vi "test variant to json uint.vi"(8 "error in (no error)":errorcluster) -> (0 "error out":errorcluster)   [LabVIEW 2019, in "labview_json_tests.lvlib"]
uses:
  labview_json_tests.lvlib
  lib/labview_json.lvlib
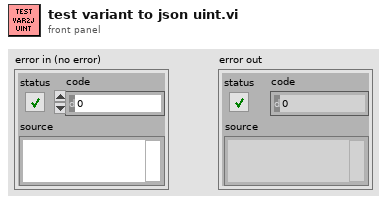
[diagram p1: front panel]
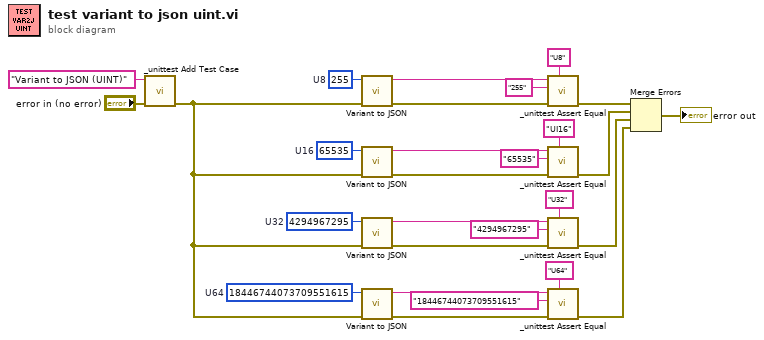
[diagram p0: block diagram]
diagram:
  w13 = u64 18446744073709551615  # U64
  w12 = u32 4294967295  # U32
  w14 = u16 65535  # U16
  w15 = u8 255  # U8
  n1 = call "_unittest Add Test Case.vi"("error in (no error)"="error in (no error)", "Test Case"="Variant to JSON (UINT)") -> ("error out"=w3:errorcluster)  [unwired: 9 in]
  n2 = call "Variant to JSON.vi"("error in (no error)"=w3, "Variant in"=w15) -> ("error out"=w21:errorcluster, "JSON"=w20:string)  [unwired: 8 in]
  n3 = call "Variant to JSON.vi"("error in (no error)"=w3, "Variant in"=w14) -> ("error out"=w19:errorcluster, "JSON"=w18:string)  [unwired: 8 in]
  n4 = call "Variant to JSON.vi"("error in (no error)"=w3, "Variant in"=w12) -> ("error out"=w6:errorcluster, "JSON"=w7:string)  [unwired: 8 in]
  n5 = call "Variant to JSON.vi"("error in (no error)"=w3, "Variant in"=w13) -> ("error out"=w8:errorcluster, "JSON"=w9:string)  [unwired: 8 in]
  n6 = call "_unittest Assert Equal.vi"("Message"="U8", "error in (no error)"=w21, "Expected Value"="255", "Actual Value"=w20) -> ("error out"=w26:errorcluster)  [unwired: 7 in]
  n7 = call "_unittest Assert Equal.vi"("Message"="UI16", "error in (no error)"=w19, "Expected Value"="65535", "Actual Value"=w18) -> ("error out"=w22:errorcluster)  [unwired: 7 in]
  n8 = call "_unittest Assert Equal.vi"("Message"="U32", "error in (no error)"=w6, "Expected Value"="4294967295", "Actual Value"=w7) -> ("error out"=w2:errorcluster)  [unwired: 7 in]
  n9 = call "_unittest Assert Equal.vi"("Message"="U64", "error in (no error)"=w8, "Expected Value"="18446744073709551615", "Actual Value"=w9) -> ("error out"=w1:errorcluster)  [unwired: 7 in]
  n10 = Merge Errors(w26, w22, w2, w1) -> (→"error out":errorcluster)
